vi "removeDevice.vi"(8 "error in (no error)":errorcluster, 10 "Remove Device in":refnum<class "IDevice.lvclass">, 11 "IDevice in":refnum<class "IDevice.lvclass">) -> (0 "error out":errorcluster, 2 "Remove Device out":refnum<class "IDevice.lvclass">, 3 "IDevice out":refnum<class "IDevice.lvclass">)   [LabVIEW 2022 SP3, in "openDAQ.lvlib" / "IBaseObject.lvlib" / "IPropertyObject.lvlib" / "IComponent.lvlib" / "IFolder.lvlib" / "IDevice.lvlib" / "IDevice.lvclass"]
uses:
  <instrlib>/openDAQ/Public/Classes/IDevice/IDevice.lvclass
  <instrlib>/openDAQ/Public/Classes/IDevice/IDevice.lvclass/IDevice.ctl
  <instrlib>/openDAQ/Binaries/Windows/x86/copendaq32.dll
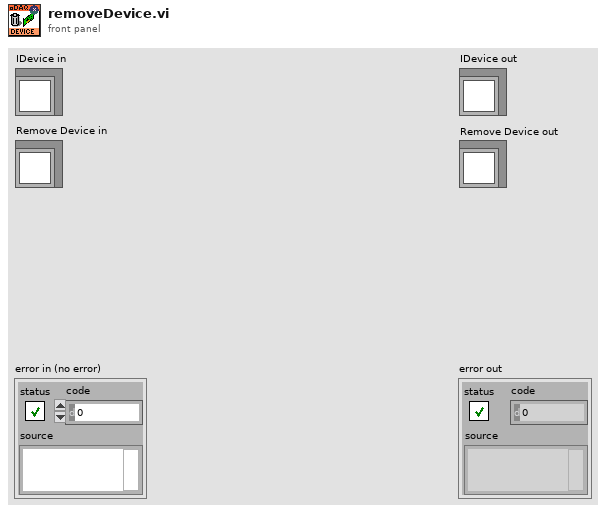
[diagram p1: front panel]
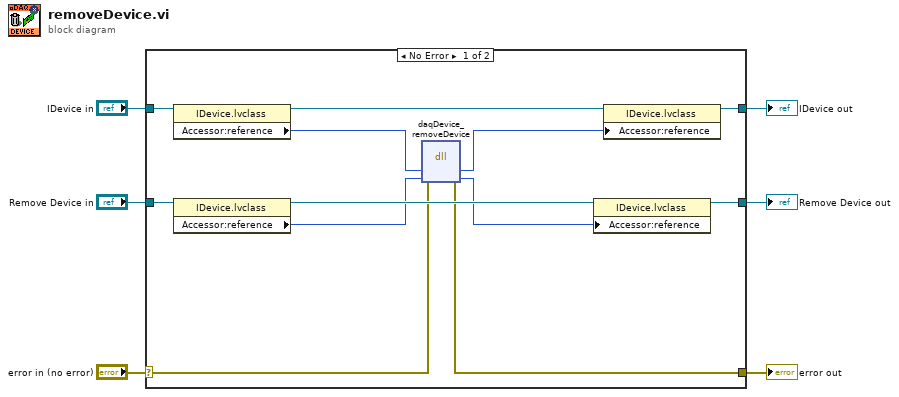
[diagram p0: block diagram]
diagram:
  n1 = case shown="No Error" "error in (no error)" {
    selector: "error in (no error)" -> [w14 w21]
    tunnel: [w13 w21] -> w5
    tunnel: [w10 w20] -> w3
    tunnel: "IDevice in" -> [w16 w20]
    tunnel: "Remove Device in" -> [w9 w19]
    tunnel: [w7 w19] -> w1
    frame No Error {
      n2 = property class="IDevice.lvclass"(reference=w16) -> (reference out=w11:refnum<class "IDevice.lvclass">, "Accessor:reference"=w15:i64)  [unwired: 1 in, 1 out]
      n3 = property class="IDevice.lvclass"(reference=w9) -> (reference out=w18:refnum<class "IDevice.lvclass">, "Accessor:reference"=w8:i64)  [unwired: 1 in, 1 out]
      n4 = dll-call lib="C:/Program Files (x86)/National Instruments/LabVIEW 2022/instr.lib/openDAQ/Binaries/Windows/x86/copendaq*.*" fn="daqDevice_removeDevice"(error in=w14, "device"=w15, "removeDevice"=w8) -> (error out=w13:errorcluster, "device"=w12:i64, "removeDevice"=w17:i64)  [unwired: 3 in, 1 out]
      n5 = property class="IDevice.lvclass"(reference=w18, "Accessor:reference"=w17) -> (reference out=w7:refnum<class "IDevice.lvclass">)  [unwired: 1 in, 1 out]
      n6 = property class="IDevice.lvclass"(reference=w11, "Accessor:reference"=w12) -> (reference out=w10:refnum<class "IDevice.lvclass">)  [unwired: 1 in, 1 out]
    }
    frame Error {
    }
  }
  "error out" <- w5
  "IDevice out" <- w3
  "Remove Device out" <- w1
